vi "save_config.vi"(2 "selected path":path, 3 "file dialog?":bool=TRUE) -> ()   [LabVIEW 2012]
doc: "Illustrates how to create and write a configuration settings file.\n\nInstructions:\nEnter values in the controls on the front panel then click on the Run Arrow.\nTo read the file, run Read Configuration Settings File.vi located in the file\\config.llb."
uses:
  global.vi
  <vilib>/Utility/config.llb/Write Key (I32).vi
  <vilib>/Utility/config.llb/Write Key (Boolean).vi
  <vilib>/Utility/config.llb/Write Key (Double).vi
  <vilib>/Utility/config.llb/Write Key (String).vi
  <vilib>/Utility/config.llb/Write Key (Path).vi
  <vilib>/Utility/config.llb/NI_LVConfig.lvlib
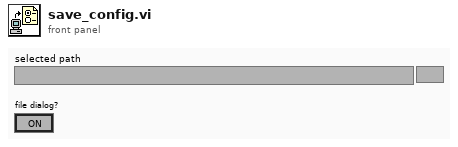
[diagram p1: front panel]
types:
  T1 = typedef "NI_LVConfig.lvlib/Config Data RefNum.ctl" = refnum<k1>
  T2 = typedef "scale.ctl" = dbl
  T3 = typedef "sampling_rate.ctl" = ext
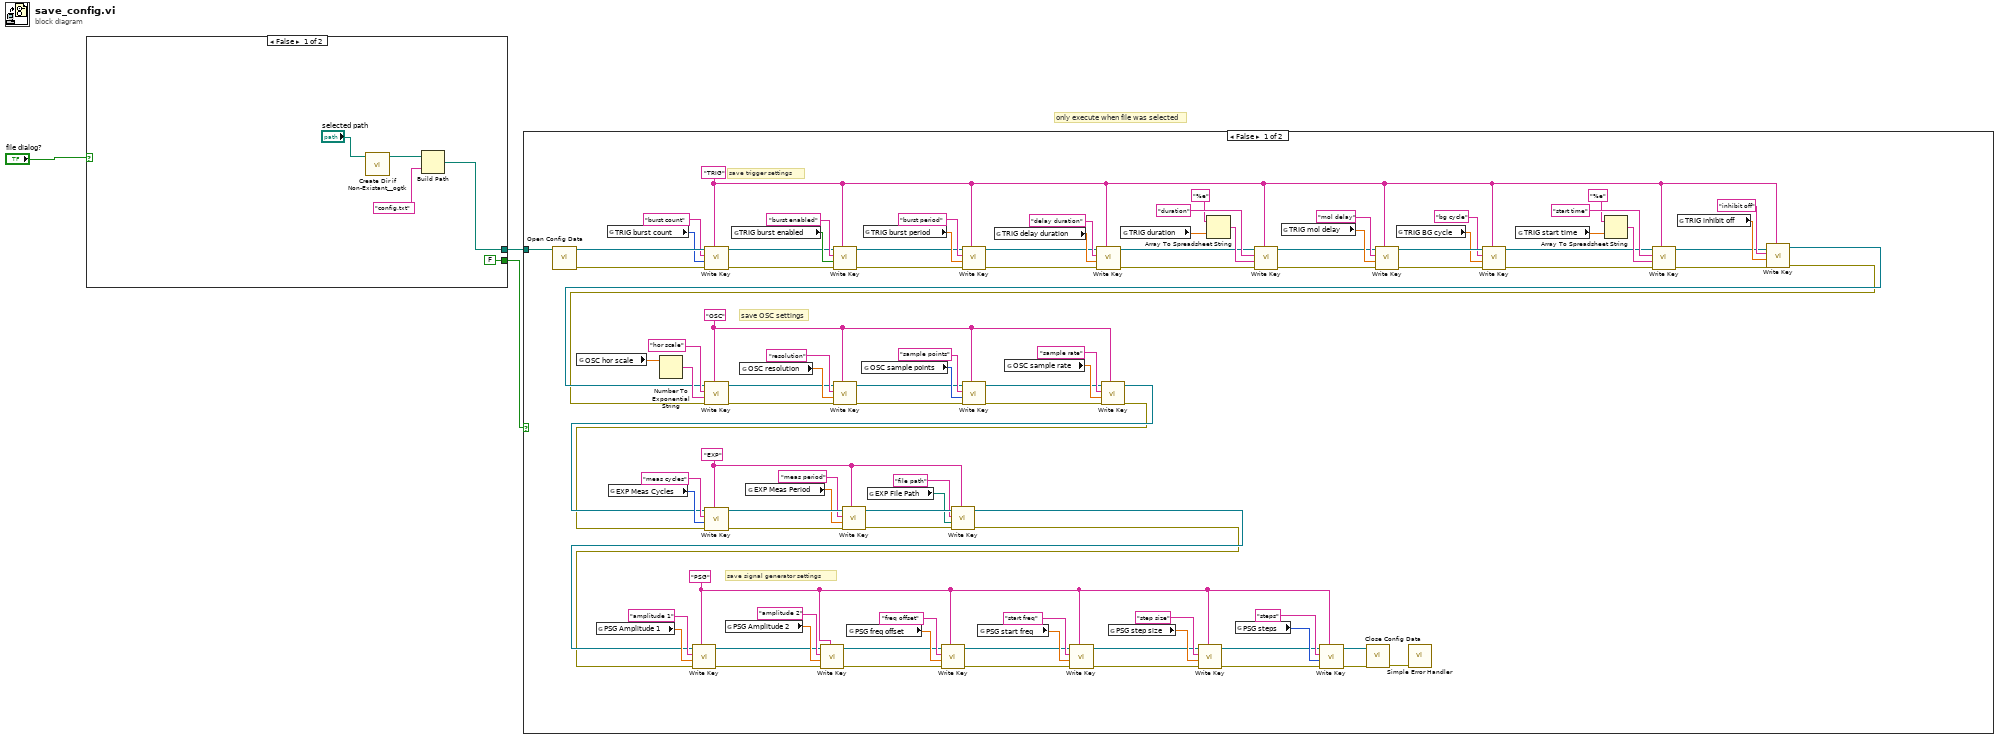
[diagram p0: block diagram]
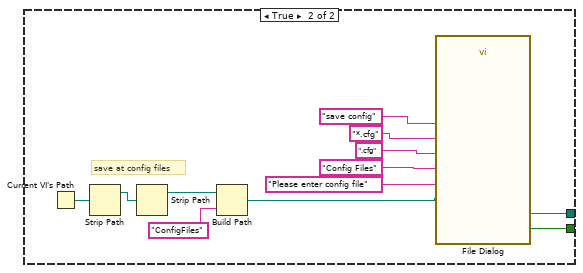
[diagram p2: hidden frame]
diagram:
  # "only execute when file was selected"
  n1 = case shown="False" "file dialog?" {
    tunnel: [w6 w20] -> w3
    tunnel: [FALSE ("cancelled") w9] -> w2
    frame False {
      n2 = call "Create Dir if Non-Existant__ogtk.vi"("Directory Path"="selected path") -> ("dup Directory Path"=w4:path)  [unwired: 8 in, 2 out]
      n3 = Build Path(base path=w4, name or relative path="config.txt") -> (appended path=w6:path)
    }
    frame True {
      # "save at config files"
      n4 = Current VI's Path() -> (path=w14:path)
      n5 = Strip Path(path=w14) -> (stripped path=w11:path)  [unwired: 1 out]
      n6 = Strip Path(path=w11) -> (stripped path=w10:path)  [unwired: 1 out]
      n7 = Build Path(base path=w10, name or relative path="ConfigFiles") -> (appended path=w12:path)
      n8 = call "File Dialog"("start path"=w12, "prompt"="Please enter config file", "button label"="save config", "default name"=".cfg", "pattern (all files)"="*.cfg", "pattern label"="Config Files") -> ("selected path"=w20:path, "cancelled"=w9:bool)  [unwired: 6 in, 2 out]
    }
  }
  n9 = case shown="False" w2 {
    tunnel: w3 -> [w117 _]
    frame False {
      w46 = "PSG"
      w23 = "EXP"
      w75 = "OSC"
      w32 = "TRIG"
      # "save signal generator settings"
      # "save OSC settings"
      # "save trigger settings"
      n10 = call <vilib>:"Open Config Data.vi"("configuration file path"=w117) -> ("error out"=w120:errorcluster, "refnum"=w121:T1)  [unwired: 2 in, 7 out]
      n11 = global read "global.vi" "OSC hor scale"() -> (w45:T2)
      n12 = global read "global.vi" "PSG Amplitude 1"() -> (w56:dbl)
      n13 = global read "global.vi" "TRIG burst count"() -> (w116:i32)
      n14 = global read "global.vi" "EXP Meas Cycles"() -> (w73:i32)
      n15 = Number To Exponential String(number=w45) -> (E-format string=w44:string)  [unwired: 3 in]
      n16 = call-poly <vilib>:"Write Key.vi"("section"=w32, "error in (no error)"=w120, "value"=w116, "key"="burst count" ("Key 1"), "refnum"=w121) -> ("error out"=w101:errorcluster, "refnum out"=w105:T1)  [unwired: 5 out]
      n17 = global read "global.vi" "PSG Amplitude 2"() -> (w54:dbl)
      n18 = global read "global.vi" "TRIG burst enabled"() -> (w114:bool)
      n19 = global read "global.vi" "OSC resolution"() -> (w86:ext)
      n20 = global read "global.vi" "EXP Meas Period"() -> (w40:dbl)
      n21 = call-poly <vilib>:"Write Key.vi"("section"=w32, "error in (no error)"=w101, "value"=w114, "key"="burst enabled" ("Key 1"), "refnum"=w105) -> ("error out"=w100:errorcluster, "refnum out"=w104:T1)  [unwired: 5 out]
      n22 = global read "global.vi" "PSG freq offset"() -> (w69:dbl)
      n23 = global read "global.vi" "OSC sample points"() -> (w84:i32)
      n24 = global read "global.vi" "TRIG burst period"() -> (w112:dbl)
      n25 = global read "global.vi" "EXP File Path"() -> (w21:path)
      n26 = call-poly <vilib>:"Write Key.vi"("section"=w32, "error in (no error)"=w100, "value"=w112, "key"="burst period" ("Key 1"), "refnum"=w104) -> ("error out"=w99:errorcluster, "refnum out"=w103:T1)  [unwired: 3 in, 2 out]
      n27 = global read "global.vi" "PSG start freq"() -> (w67:dbl)
      n28 = global read "global.vi" "TRIG delay duration"() -> (w110:dbl)
      n29 = global read "global.vi" "OSC sample rate"() -> (w78:T3)
      n30 = call-poly <vilib>:"Write Key.vi"("section"=w32, "error in (no error)"=w99, "value"=w110, "key"="delay duration" ("Key 1"), "refnum"=w103) -> ("error out"=w98:errorcluster, "refnum out"=w102:T1)  [unwired: 3 in, 2 out]
      n31 = global read "global.vi" "PSG step size"() -> (w65:dbl)
      n32 = global read "global.vi" "TRIG duration"() -> (w107:dbl[])
      n33 = Array To Spreadsheet String(array=w107, 3:"%e" ("format string")) -> (spreadsheet string=w106:string)  [unwired: 1 in]
      n34 = global read "global.vi" "PSG steps"() -> (w59:i32)
      n35 = call-poly <vilib>:"Write Key.vi"("section"=w32, "error in (no error)"=w98, "value"=w106, "key"="duration" ("Key 1"), "refnum"=w102) -> ("error out"=w90:errorcluster, "refnum out"=w91:T1)  [unwired: 1 in, 4 out]
      n36 = global read "global.vi" "TRIG mol delay"() -> (w92:dbl)
      n37 = call-poly <vilib>:"Write Key.vi"("section"=w32, "error in (no error)"=w90, "value"=w92, "key"="mol delay" ("Key 1"), "refnum"=w91) -> ("error out"=w89:errorcluster, "refnum out"=w38:T1)  [unwired: 3 in, 2 out]
      n38 = global read "global.vi" "TRIG BG cycle"() -> (w35:dbl)
      n39 = call-poly <vilib>:"Write Key.vi"("section"=w32, "error in (no error)"=w89, "value"=w35, "key"="bg cycle" ("Key 1"), "refnum"=w38) -> ("error out"=w39:errorcluster, "refnum out"=w37:T1)  [unwired: 4 in, 1 out]
      n40 = global read "global.vi" "TRIG start time"() -> (w95:dbl[])
      n41 = Array To Spreadsheet String(array=w95, 3:"%e" ("format string")) -> (spreadsheet string=w94:string)  [unwired: 1 in]
      n42 = call-poly <vilib>:"Write Key.vi"("section"=w32, "error in (no error)"=w39, "value"=w94, "key"="start time" ("Key 1"), "refnum"=w37) -> ("error out"=w29:errorcluster, "refnum out"=w31:T1)  [unwired: 1 in, 4 out]
      n43 = global read "global.vi" "TRIG inhibit off"() -> (w34:dbl)
      n44 = call-poly <vilib>:"Write Key.vi"("section"=w32, "error in (no error)"=w29, "value"=w34, "key"="inhibit off" ("Key 1"), "refnum"=w31) -> ("error out"=w28:errorcluster, "refnum out"=w30:T1)  [unwired: 3 in, 2 out]
      n45 = call-poly <vilib>:"Write Key.vi"("section"=w75, "error in (no error)"=w28, "value"=w44, "key"="hor scale" ("Key 1"), "refnum"=w30) -> ("error out"=w81:errorcluster, "refnum out"=w83:T1)  [unwired: 1 in, 4 out]
      n46 = call-poly <vilib>:"Write Key.vi"("section"=w75, "error in (no error)"=w81, "value"=w86, "key"="resolution" ("Key 1"), "refnum"=w83) -> ("error out"=w80:errorcluster, "refnum out"=w82:T1)  [unwired: 3 in, 2 out]
      n47 = call-poly <vilib>:"Write Key.vi"("section"=w75, "error in (no error)"=w80, "value"=w84, "key"="sample points" ("Key 1"), "refnum"=w82) -> ("error out"=w76:errorcluster, "refnum out"=w77:T1)  [unwired: 5 out]
      n48 = call-poly <vilib>:"Write Key.vi"("section"=w75, "error in (no error)"=w76, "value"=w78, "key"="sample rate" ("Key 1"), "refnum"=w77) -> ("error out"=w71:errorcluster, "refnum out"=w72:T1)  [unwired: 3 in, 2 out]
      n49 = call-poly <vilib>:"Write Key.vi"("section"=w23, "error in (no error)"=w71, "value"=w73, "key"="meas cycles" ("Key 1"), "refnum"=w72) -> ("error out"=w42:errorcluster, "refnum out"=w43:T1)  [unwired: 5 out]
      n50 = call-poly <vilib>:"Write Key.vi"("section"=w23, "error in (no error)"=w42, "value"=w40, "key"="meas period" ("Key 1"), "refnum"=w43) -> ("error out"=w26:errorcluster, "refnum out"=w27:T1)  [unwired: 3 in, 2 out]
      n51 = call-poly <vilib>:"Write Key.vi"("section"=w23, "error in (no error)"=w26, "value"=w21, "key"="file path" ("Key 1"), "refnum"=w27) -> ("error out"=w24:errorcluster, "refnum out"=w25:T1)  [unwired: 5 out]
      n52 = call-poly <vilib>:"Write Key.vi"("section"=w46, "error in (no error)"=w24, "value"=w56, "key"="amplitude 1" ("Key 1"), "refnum"=w25) -> ("error out"=w52:errorcluster, "refnum out"=w53:T1)  [unwired: 3 in, 2 out]
      n53 = call-poly <vilib>:"Write Key.vi"("section"=w46, "error in (no error)"=w52, "value"=w54, "key"="amplitude 2" ("Key 1"), "refnum"=w53) -> ("error out"=w51:errorcluster, "refnum out"=w50:T1)  [unwired: 3 in, 2 out]
      n54 = call-poly <vilib>:"Write Key.vi"("section"=w46, "error in (no error)"=w51, "value"=w69, "key"="freq offset" ("Key 1"), "refnum"=w50) -> ("error out"=w62:errorcluster, "refnum out"=w64:T1)  [unwired: 3 in, 2 out]
      n55 = call-poly <vilib>:"Write Key.vi"("section"=w46, "error in (no error)"=w62, "value"=w67, "key"="start freq" ("Key 1"), "refnum"=w64) -> ("error out"=w61:errorcluster, "refnum out"=w63:T1)  [unwired: 3 in, 2 out]
      n56 = call-poly <vilib>:"Write Key.vi"("section"=w46, "error in (no error)"=w61, "value"=w65, "key"="step size" ("Key 1"), "refnum"=w63) -> ("error out"=w57:errorcluster, "refnum out"=w58:T1)  [unwired: 3 in, 2 out]
      n57 = call-poly <vilib>:"Write Key.vi"("section"=w46, "error in (no error)"=w57, "value"=w59, "key"="steps" ("Key 1"), "refnum"=w58) -> ("error out"=w48:errorcluster, "refnum out"=w49:T1)  [unwired: 5 out]
      n58 = call <vilib>:"Close Config Data.vi"("error in (no error)"=w48, "refnum"=w49) -> ("error out"=w118:errorcluster)  [unwired: 1 in, 8 out]
      n59 = call <vilib>:"Simple Error Handler.vi"("error in (no error)"=w118) -> ()  [unwired: 1 in, 8 out]
    }
    frame True {
    }
  }
